vi "Test Mode and Write.vi"(8 "Error In":errorcluster) -> (0 "Error Out":errorcluster)   [LabVIEW 2014, in "STM32F4 Discovery General Wrapper.lvlib"]
uses:
  <vilib>/Aledyne-TSXperts/Arduino Compatible Compiler for LabVIEW/addons/STM32F4 Discovery General Wrapper/STM32F4 Discovery General Wrapper.lvlib
  <vilib>/Aledyne-TSXperts/Arduino Compatible Compiler for LabVIEW/addons/STM32F4 Discovery General Wrapper/Ctl/PinList.ctl
  <vilib>/Aledyne-TSXperts/Arduino Compatible Compiler for LabVIEW/addons/STM32F4 Discovery General Wrapper/Ctl/PinModes.ctl
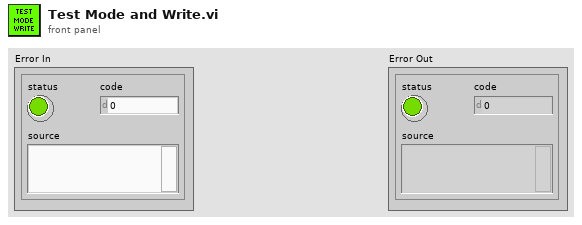
[diagram p1: front panel]
types:
  T1 = typedef "STM32F4 Discovery General Wrapper.lvlib/PinModes.ctl" = enum16{"OUTPUT", "OUTPUT_OPEN_DRAIN", "INPUT", "INPUT_ANALOG", "INPUT_PULLUP", "INPUT_PULLDOWN", "INPUT_FLOATING", "PWM", "PWM_OPEN_DRAIN"}
  T2 = typedef "STM32F4 Discovery General Wrapper.lvlib/PinList.ctl" = enum8{"PA0", "PA1", "PA2", "PA3", "PA4", "PA5", "PA6", "PA7", "PA8", "PA9", "PA10", "PA11", "PA12", "PA13", "PA14", "PA15", "PB0", "PB1", "PB2", "PB3", "PB4", "PB5", "PB6", "PB7", "PB8", "PB9", "PB10", "PB11", "PB12", "PB13", "PB14", "PB15", "PC0", "PC1", "PC2", "PC3", "PC4", "PC5", "PC6", "PC7", "PC8", "PC10", "PC11", "PC12", "PC13", "PC14", "PC15", "PD0", "PD1", "PD2", "PD3", "PD4", "PD5", "PD6", "PD7", "PD8", "PD9", "PD10", "PD11", "PD12", "PD13", "PD14", "PD15", "PE0", "PE1", "PE2", "PE3", "PE4", "PE5", "PE6", "PE7", "PE8", "PE9", "PE10", "PE11", "PE12", "PE13", "PE14", "PE15", "PF0", "PF1", "PF2", "PF3", "PF4", "PF5", "PF6", "PF7", "PF8", "PF9", "PF10", "PF11", "PF12", "PF13", "PF14", "PF15", "PG0", "PG1", "PG2", "PG3", "PG4", "PG5", "PG6", "PG7", "PG8", "PG9", "PG10", "PG11", "PG12", "PG13", "PG14", "PG15"}
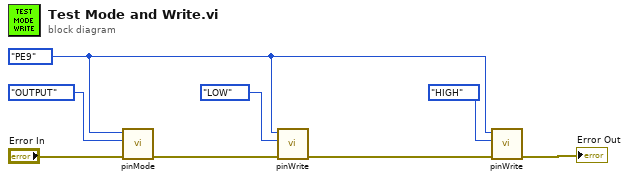
[diagram p0: block diagram]
diagram:
  w6 = PinList."PE9" ("Pin number")
  n1 = call <vilib>:"pinMode.vi"("Error In"="Error In", "Pin mode"=PinModes."OUTPUT", "Pin number"=w6) -> ("Error Out"=w8:errorcluster)  [unwired: 8 in]
  n2 = call <vilib>:"pinWrite.vi"("Error In"=w8, "State 2"=enum16{"LOW", "HIGH"}."LOW", "Pin number"=w6) -> ("Error Out"=w2:errorcluster)  [unwired: 8 in]
  n3 = call <vilib>:"pinWrite.vi"("Error In"=w2, "State 2"=enum16{"LOW", "HIGH"}."HIGH", "Pin number"=w6) -> ("Error Out"=→"Error Out":errorcluster)  [unwired: 8 in]
